vi "VDH-RequestCalibrateSOLT.vi"(8 "error in (no error)":errorcluster, 10 "SOLT":T1=enum."Short", 11 "VDH-VNA_data_handler in":refnum<class "VDH-VNA_data_handler.lvclass">) -> (0 "error out":errorcluster, 3 "VDH-VNA_data_handler out":refnum<class "VDH-VNA_data_handler.lvclass">)   [LabVIEW 2020, in "VDH-VNA_data_handler.lvlib" / "VDH-VNA_data_handler.lvclass"]
uses:
  VDH-VNA_data_handler.lvclass
  VDH-Calibration_enum.ctl
  VDH-Calibration_temp_storage.ctl
  VDH-VNA_data_handler.lvclass/VDH-VNA_data_handler.ctl
  hardware_manager/VHM-VNA_Hardware_Manager/VHM-VNA_Hardware_Manager Messages/VHM-getDataSet Msg/VHM-getDataSet Msg.lvclass
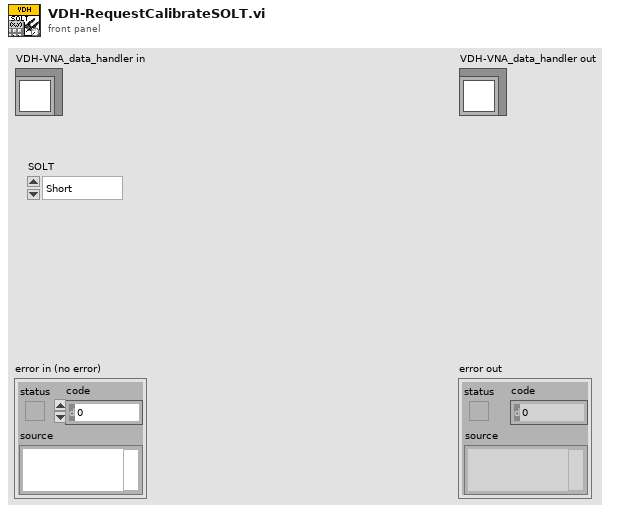
[diagram p1: front panel]
types:
  T1 = typedef "VDH-VNA_data_handler.lvlib/VDH-VNA_data_handler.lvclass/VDH-Calibration_enum.ctl" = enum16{"Non", "Short", "Open", "Load", "Through", "Permativity"}
  T2 = typedef "VDH-VNA_data_handler.lvlib/VDH-VNA_data_handler.lvclass/VDH-Calibration_temp_storage.ctl" = cluster{"S11":cdb[][]}
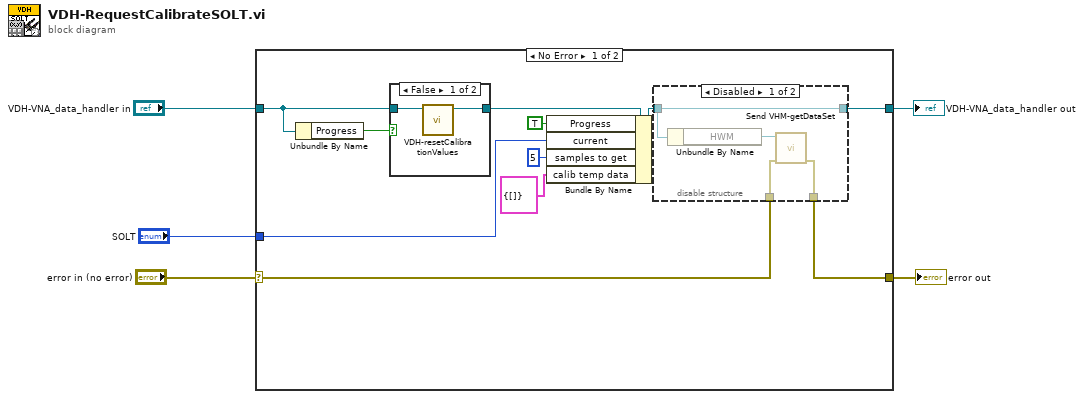
[diagram p0: block diagram]
diagram:
  n1 = case shown="No Error" "error in (no error)" {
    selector: "error in (no error)" -> [w10 w27]
    tunnel: [w9 w27] -> w4
    tunnel: [w7 w26] -> w2
    tunnel: "VDH-VNA_data_handler in" -> [w15 w26]
    tunnel: "SOLT" -> [w12 _]
    frame No Error {
      n2 = Unbundle By Name(w15) -> ("Progress"=w16:bool)
      n3 = case shown="False" w16 {
        tunnel: w15 -> [w24 w25]
        tunnel: [w23 w25] -> w14
        frame False {
          n4 = call "VDH-resetCalibrationValues.vi"("VDH-VNA_data_handler in"=w24) -> ("VDH-VNA_data_handler out"=w23:refnum<class "VDH-VNA_data_handler.lvclass">)  [unwired: 10 in]
        }
        frame True {
        }
      }
      n5 = Bundle By Name(cluster=w14, "Progress"=TRUE ("Calibration Status.Progress.Progress"), "current"=w12, "samples to get"=u8 5 ("Calibration Status.Progress.samples to get"), "calib temp data"=T2 {"S11"=[]}) -> (w11:refnum<class "VDH-VNA_data_handler.lvclass">)
      n6 = disable-structure shown="Disabled" {
        disable-tunnel: w11 -> [w17 w21]
        disable-tunnel: w10 -> [w19 w22]
        disable-tunnel: [w18 w22] -> w9
        disable-tunnel: [w17 w21] -> w7
        frame Disabled {
          n7 = Unbundle By Name(w17) -> ("HWM"=w20:refnum<class "Message Enqueuer.lvclass">)
          n8 = call "Send VHM-getDataSet.vi"("error in (no error)"=w19, "Message Enqueuer"=w20) -> ("error out"=w18:errorcluster)  [unwired: 8 in, 1 out]
        }
        frame Enabled {
        }
      }
    }
    frame Error {
    }
  }
  "error out" <- w4
  "VDH-VNA_data_handler out" <- w2
